vi "GetAllPPLFunction_VisionAnalysis.vi"() -> (2 "PluginRunTime Folder":path, 3 "AnalysisFunction":string[](array[string]))   [LabVIEW 2019]
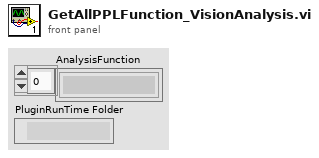
[diagram p1: front panel]
types:
  T1 = enum32{"invalid app kind", "Development System", "Run Time System", "Student Edition", "Embedded LabVIEW", "Evaluation", "Custom"}
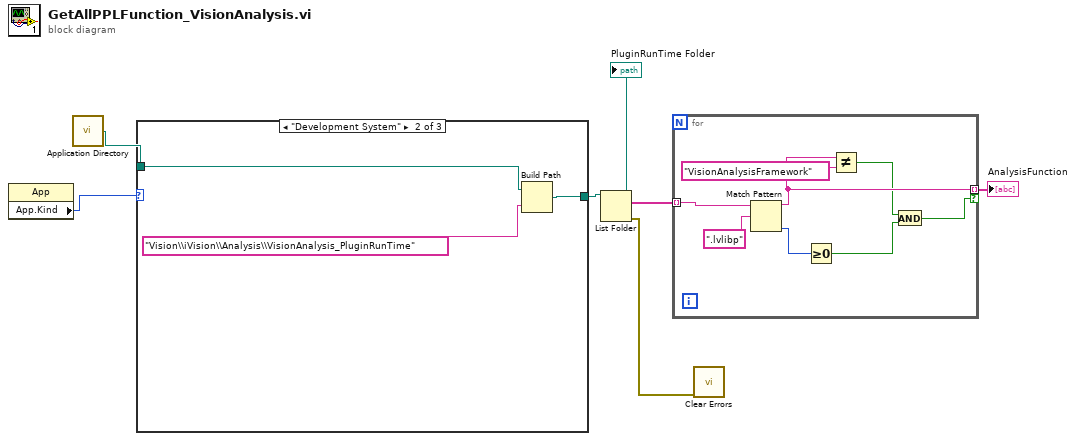
[diagram p0: block diagram]
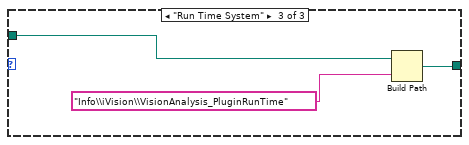
[diagram p3: hidden frame]
diagram:
  n1 = property class="App"() -> ("App.Kind"=w6:T1)  [unwired: 2 in, 2 out]
  n2 = call <vilib>:"Application Directory.vi"() -> ("Application Directory"=w5:path)
  n3 = case shown="\"Development System\"" w6 {
    tunnel: [_ w9 w12] -> w4
    tunnel: w5 -> [_ w8 w11]
    frame "invalid app kind", Default {
    }
    frame "Development System" {
      n4 = Build Path(base path=w8, name or relative path="Vision\\iVision\\Analysis\\VisionAnalysis_PluginRunTime") -> (appended path=w9:path)
    }
    frame "Run Time System" {
      n5 = Build Path(base path=w11, name or relative path="Info\\iVision\\VisionAnalysis_PluginRunTime") -> (appended path=w12:path)
    }
  }
  "PluginRunTime Folder" <- w4
  n6 = List Folder(path=w4) -> (filenames=w3:string[], error out=w1:errorcluster)  [unwired: 3 in, 2 out]
  n7 = for {
    tunnel: w3 -> [w18] mode=indexing
    tunnel: [w17] -> w2 mode=indexing if=w13
    n8 = Match Pattern(string=w18, regular expression=".lvlibp") -> (before substring=w17:string, offset past match=w19:i32)  [unwired: 1 in, 2 out]
    n9 = Greater Or Equal To 0?(x=w19) -> (x >= 0?=w14:bool)
    n10 = Not Equal?(x=w17, y="VisionAnalysisFramework") -> (x != y?=w15:bool)
    n11 = And(x=w15, y=w14) -> (x .and. y?=w13:bool)
  }
  "AnalysisFunction" <- w2
  n12 = call <vilib>:"Clear Errors.vi"("error in (no error)"=w1) -> ()  [unwired: 5 in, 2 out]
